vi "Append unique suffix.vi"(6 "Extention":string, 7 "Suffix":string, 8 "error in (no error)":errorcluster, 11 "Path":path) -> (0 "error out":errorcluster, 3 "Path out":path)   [LabVIEW 2019]
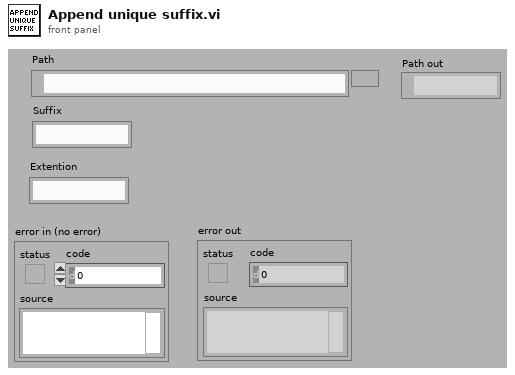
[diagram p1: front panel]
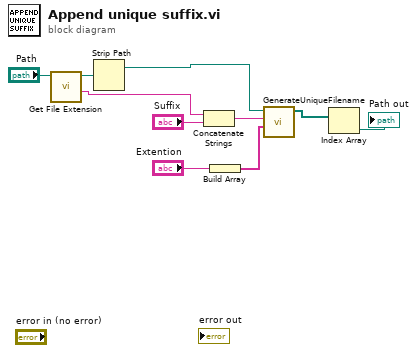
[diagram p0: block diagram]
diagram:
  n1 = call <vilib>:"Get File Extension.vi"("file"="Path") -> ("filename without extension"=w4:string, "dup file"=w3:path)  [unwired: 6 in, 3 out]
  n2 = Strip Path(path=w3) -> (stripped path=w6:path)  [unwired: 1 out]
  n3 = Concatenate Strings(w4, "Suffix") -> (w9:string)
  n4 = Build Array("Extention") -> (w7:string[])
  n5 = call "GenerateUniqueFilename.vi"("File name suffixes"=w7, "File name prefix"=w9, "Folder Path Control"=w6) -> ("Paths"=w2:path[])  [unwired: 7 in, 1 out]
  n6 = Index Array(array=w2) -> (element=→"Path out":path)  [unwired: 1 in]
